vi "generate_header.vi"() -> (3 "header\narray":string[](array[string]))   [LabVIEW 2018]
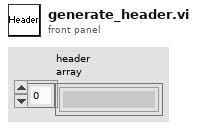
[diagram p1: front panel]
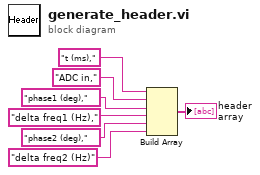
[diagram p0: block diagram]
diagram:
  n1 = Build Array("t (ms),", "ADC in,", "phase1 (deg),", "delta freq1 (Hz),", "phase2 (deg),", "delta freq2 (Hz)") -> (→"header\narray":string[])
